vi "Dashboard Main.vi"() -> ()   [LabVIEW 2020]
uses:
  <vilib>/Utility/miscctls.llb/LVRowAndColumnTypeDef.ctl
  <vilib>/event_ctls.llb/eventvkey.ctl
  <vilib>/Rock Robotics/Network Tables/NT Read Numeric Array.vi
  <vilib>/Rock Robotics/Network Tables/NT Read Boolean.vi
  <vilib>/Rock Robotics/WPI/Dashboard/WPI_DashboardLogging Global.vi
panel:
  in  "Camera Settings Right":T1={"Frame Rate"=30, "Compression"=30, "Size"=1, "DB Camera Config"=FALSE} {"Frame Rate" scale=1.0..30.0; "Compression" scale=100.0..-1.0; "Size" items=["640x480", "320x240", "160x120"]}
  in  "Camera Name Right":string(combo)="No Camera Selection"
  out "Camera Perf":string
  in  "Camera Settings":T1={"Frame Rate"=30, "Compression"=30, "Size"=1, "DB Camera Config"=FALSE} {"Frame Rate" scale=1.0..30.0; "Compression" scale=100.0..-1.0; "Size" items=["640x480", "320x240", "160x120"]}
  in  "TCP":refnum<k5>
  in  "Rec Mode":enum32{"Stop", "Record", "Playback"}(radio)
  out "Robot IP":string
  out "Image Message":string="Timeout in Camera Communications"
  in  "Dashboard Tab":T2(tab)
  in  "Select Auto":string(combo)="Select Autonomous ..."
  out "NT Connection":bool
  out "MotorChart R":cluster{"Numeric":dbl, "Numeric":dbl}(graph)
  out "MotorChart L":cluster{"Numeric":dbl, "Numeric":dbl}(graph)
  out "MotorSliders R":cluster{"MotorSlide1":dbl, "MotorSlide2":dbl} {"MotorSlide2" scale=-1.0..1.0 scale format="%#_2e"; "MotorSlide1" scale=-1.0..1.0 scale format="%#_2e"}
  out "MotorSliders L":cluster{"MotorSlide1":dbl, "MotorSlide2":dbl} {"MotorSlide2" scale=-1.0..1.0 scale format="%#_2e"; "MotorSlide1" scale=-1.0..1.0 scale format="%#_2e"}
  out "Gyro":dbl(knob) scale=0.0..360.0
  out "JS1 Z":dbl(slide) scale=-1.0..1.0 scale format="%#_2e"
  out "JS1 Graph":cluster{"X":dbl, "Y":dbl}[](graph)
  out "JS1 Buttons":T3
  out "JS2 Z":dbl(slide) scale=-1.0..1.0 scale format="%#_2e"
  out "JS2 Graph":cluster{"X":dbl, "Y":dbl}[](graph)
  out "JS2 Buttons":T3
  out "Mode":T4(ring)=enum."Auto Disabled"
  out "Right Camera Perf":cluster{"Bandwidth (Mbps)":dbl, "FPS":dbl}
  out "Camera Image Right":T5(plugin-control)
  in  "DB/String 9":string
  in  "DB/String 8":string
  in  "DB/String 7":string
  in  "DB/String 6":string
  in  "DB/String 5":string
  in  "DB/String 4":string
  in  "DB/String 3":string
  in  "DB/String 2":string
  in  "DB/String 1":string
  in  "DB/String 0":string
  in  "DB/Slider 0":dbl(slide) scale=0.0..5.0
  in  "DB/Slider 1":dbl(slide) scale=0.0..5.0
  in  "DB/Slider 2":dbl(slide) scale=0.0..5.0
  in  "DB/Slider 3":dbl(slide) scale=0.0..5.0
  out "DB/LED 3":bool
  out "DB/LED 2":bool
  out "DB/LED 1":bool
  out "DB/LED 0":bool
  in  "DB/Button 3":bool
  in  "DB/Button 2":bool
  in  "DB/Button 1":bool
  in  "DB/Button 0":bool caption="New Name"
  out "Climb Time":dbl
  out "Current Shot":string
  out "Locked On":bool
  out "Ball Count":i32(slide) scale=0.0..2.0
  in  "Autonomous Selector":string(combo)
  in  "Test Slider":dbl(slide) scale=0.0..100.0 scale format="%#_3g"
  in  "On/Off":bool caption="Solenoid"
  in  "Test Name":u16(ring) items=["Select the test to run..."]
  in  "Test Tree":string(tree)
  in  "Motor":cluster{"Value":dbl, "Enable":bool} {"Value" scale=-1.0..1.0 scale format="%#_3g"}
  out "Progress":T6 {"Test Progress" scale=0.0..100.0}
  in  "Rev/Fwd":cluster{"Forward":bool, "Reverse":bool}
  in  "Test Ring":u16(ring) items=["Monochrome", "Color"]
  out "Cmd Status":string
  in  "Execute Command":bool
  in  "Command Params":string[][](table)
  in  "Command Selection":i32(listbox)
  in  "CheckList":i32(listbox)
  out "Tree":string(tree)
  out "Camera Image":T5(plugin-control)
  out "Background":bool
  in  "Camera Name":string(combo)="No Camera Selection"
  # "HW"
  # "HW"
  # "Joysticks"
  # "Drive Motors"
  # "Front"
  # "Right"
  # "Left"
  # "Back"
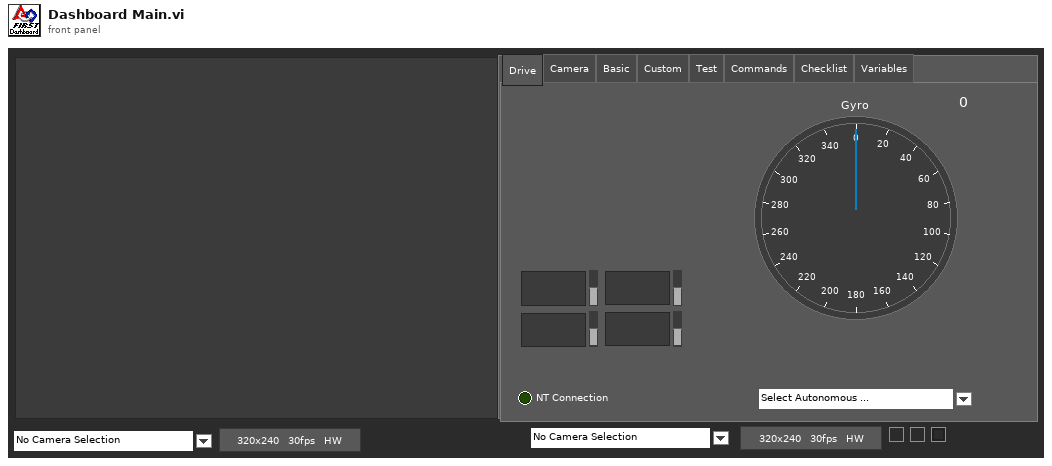
[diagram p1: front panel]
types:
  T1 = cluster{"Frame Rate":i32, "Compression":i32, "Size":u16, "DB Camera Config":bool}
  T2 = enum32{"Drive", "Camera", "Basic", "Custom", "Test", "Commands", "Checklist", "Variables"}
  T3 = cluster{bool, bool, bool, bool, bool, bool, bool, bool, bool, bool, bool, bool}
  T4 = enum8{"Tele-Op Disabled", "Tele-Op Enabled", "Auto Disabled", "Auto Enabled", "Test Disabled", "Test Enabled", "Disconnected", "No Code", "E-Stop"}
  T5 = typedef "IMAQ Image.ctl" = refnum<image>
  T6 = cluster{"Test Progress":u8, "Test Progress Text":string}
  T7 = cluster{"Save Path":path, "Interval (s)":dbl, "Keep":i32}
  T8 = typedef "Image Type" = u32
  T9 = cluster{"IDs":cluster{"RPC field ID":u16, "Unique ID":u16}, "String":string}
  T10 = cluster{"Error Strings":string, "Disable Counts":cluster{u16, u16}, "Rail Faults":cluster{u16, u16, u16}, "Robot IP":string, "DB Mode":u8, "Event Info":cluster{"Name":string, "Type":u8, "Number":u16, "Replay":u8}}
  T11 = cluster{"Storage":cluster{"Disk Free":u64, "RAM Block":u32, "RAM free":u32}, "CPU Utilization":cluster{"CPU % ISR":sgl, "CPU % Time Crit":sgl, "CPU % Timed Str":sgl, "CPU % High":sgl, "CPU % Above":sgl, "CPU % Normal":sgl, "CPU % Low":sgl}, "CAN":cluster{"% Bus Utilization":sgl, "Bus Off Cnt":u32, "TX_FIFO Full Cnt":u32, "Receive Error Cnt":u8, "Transmit Error Cnt":u8}, "HID":cluster{"HID Outputs":u32, "Rumble Low":u16, "Rumble High":u16}[]}
  T12 = cluster{"Status bits":cluster{"Test Mode":bool, "Autonomous":bool, "Enabled":bool, "Code Start":bool, "Brownout":bool, "Reserved 2":bool, "Reserved 3":bool, "E-Stop":bool}, "Code Trace":cluster{"Disabled":bool, "TeleOp":bool, "Auto":bool, "Test":bool}, "Controller Type":enum16{"unknown", "cRIO", "roboRio"}, "Code?":enum16{"unknown", "noCode", "code"}, "Battery V":dbl}
  T13 = cluster{"Control Bits":cluster{"TestMode":bool, "Autonomous":bool, "Enabled":bool, "FMS Present":bool, bool, bool, bool, "E-Stop":bool}, "Team Station ":u8, "Countdown":sgl, "Joystick Values":cluster{"Axes":dbl[], "Buttons":bool[], "POVs":i16[]}[]}
  T14 = cluster{"Axes":dbl[], "Buttons":bool[], "POVs":i16[]}[]
  T15 = cluster{"Axes":dbl[], "Buttons":bool[], "POVs":i16[]}
  T16 = cluster{"Buttons[0]":bool, "Buttons[1]":bool, "Buttons[2]":bool, "Buttons[3]":bool, "Buttons[4]":bool, "Buttons[5]":bool, "Buttons[6]":bool, "Buttons[7]":bool, "Buttons[8]":bool, "Buttons[9]":bool, "Buttons[10]":bool, "Buttons[11]":bool}
  T17 = cluster{"Camera Image":refnum<vi>, "Dashboard Tab":refnum<vi>, "Background":refnum<vi>, "Rec Mode":refnum<vi>, "Test Slider":refnum<vi>, "On/Off ":refnum<vi>, "Test Ring":refnum<vi>, "Rev/Fwd":refnum<vi>, "Test Name":refnum<vi>, "Motor":refnum<vi>, "Progress":refnum<vi>, "CheckList":refnum<vi>, "Tree":refnum<vi>, "Test Tree":refnum<vi>, "Command Params":refnum<vi>, "Command Selection":refnum<vi>, "Execute Command":refnum<vi>, "Cmd Status":refnum<vi>, "Camera Settings":refnum<vi>, "Camera Name":refnum<vi>, "Camera Perf":refnum<vi>, "Camera Settings Right":refnum<vi>, "Camera Name Right":refnum<vi>, "Camera Image Right":refnum<vi>}
  T18 = cluster{"Global Rectangle":i32[], "Contours":cluster{"Contour Type":u32, "ROI Type":u32, "Points":i32[]}[]}
  T19 = cluster{"Camera Name":string, string, "Saved DB Images Info":cluster{"Save Path":path, "Interval (s)":dbl, "Keep":i32}}
  T20 = cluster{"Camera Name Right":string, string, "Saved DB Images Info":cluster{"Save Path":path, "Interval (s)":dbl, "Keep":i32}}
  T21 = cluster{"Operation":enum16{"Update", "Clear"}, "Color Box":u32}[]
  T22 = typedef "eventvkey.ctl" = enum16{"ASCII", "Enter", "Return", "Shift", "Ctrl", "Alt", "Cmd", "Opt", "Caps", "NumLock", "Clear", "Break", "Up", "Down", "Left", "Right", "Insert", "Delete", "Home", "End", "PageUp", "PageDown", "Escape", "Help", "Pause", "ScrollLock", "F1", "F2", "F3", "F4", "F5", "F6", "F7", "F8", "F9", "F10", "F11", "F12", "F13", "F14", "F15", "F16", "F17", "F18", "F19", "F20", "F21", "F22", "F23", "F24", "Play", "VolumeUp", "VolumeDown", "Mute", "Two Byte Char"}
  T23 = cluster{"Image Size":bool, "Image Type":bool, "Pixel Value":bool, "ROI Information":bool, "Zoom Factor":bool}
  T24 = cluster{"Operation":enum16{"Update", "Clear"}, "Color Box":u32}
  T25 = typedef "LVRowAndColumnTypeDef.ctl" = cluster{"Row":i32, "Column":i32}
  T26 = cluster{"Shift":bool, "Ctrl":bool, "Alt":bool, "Cmd":bool, "Opt":bool}
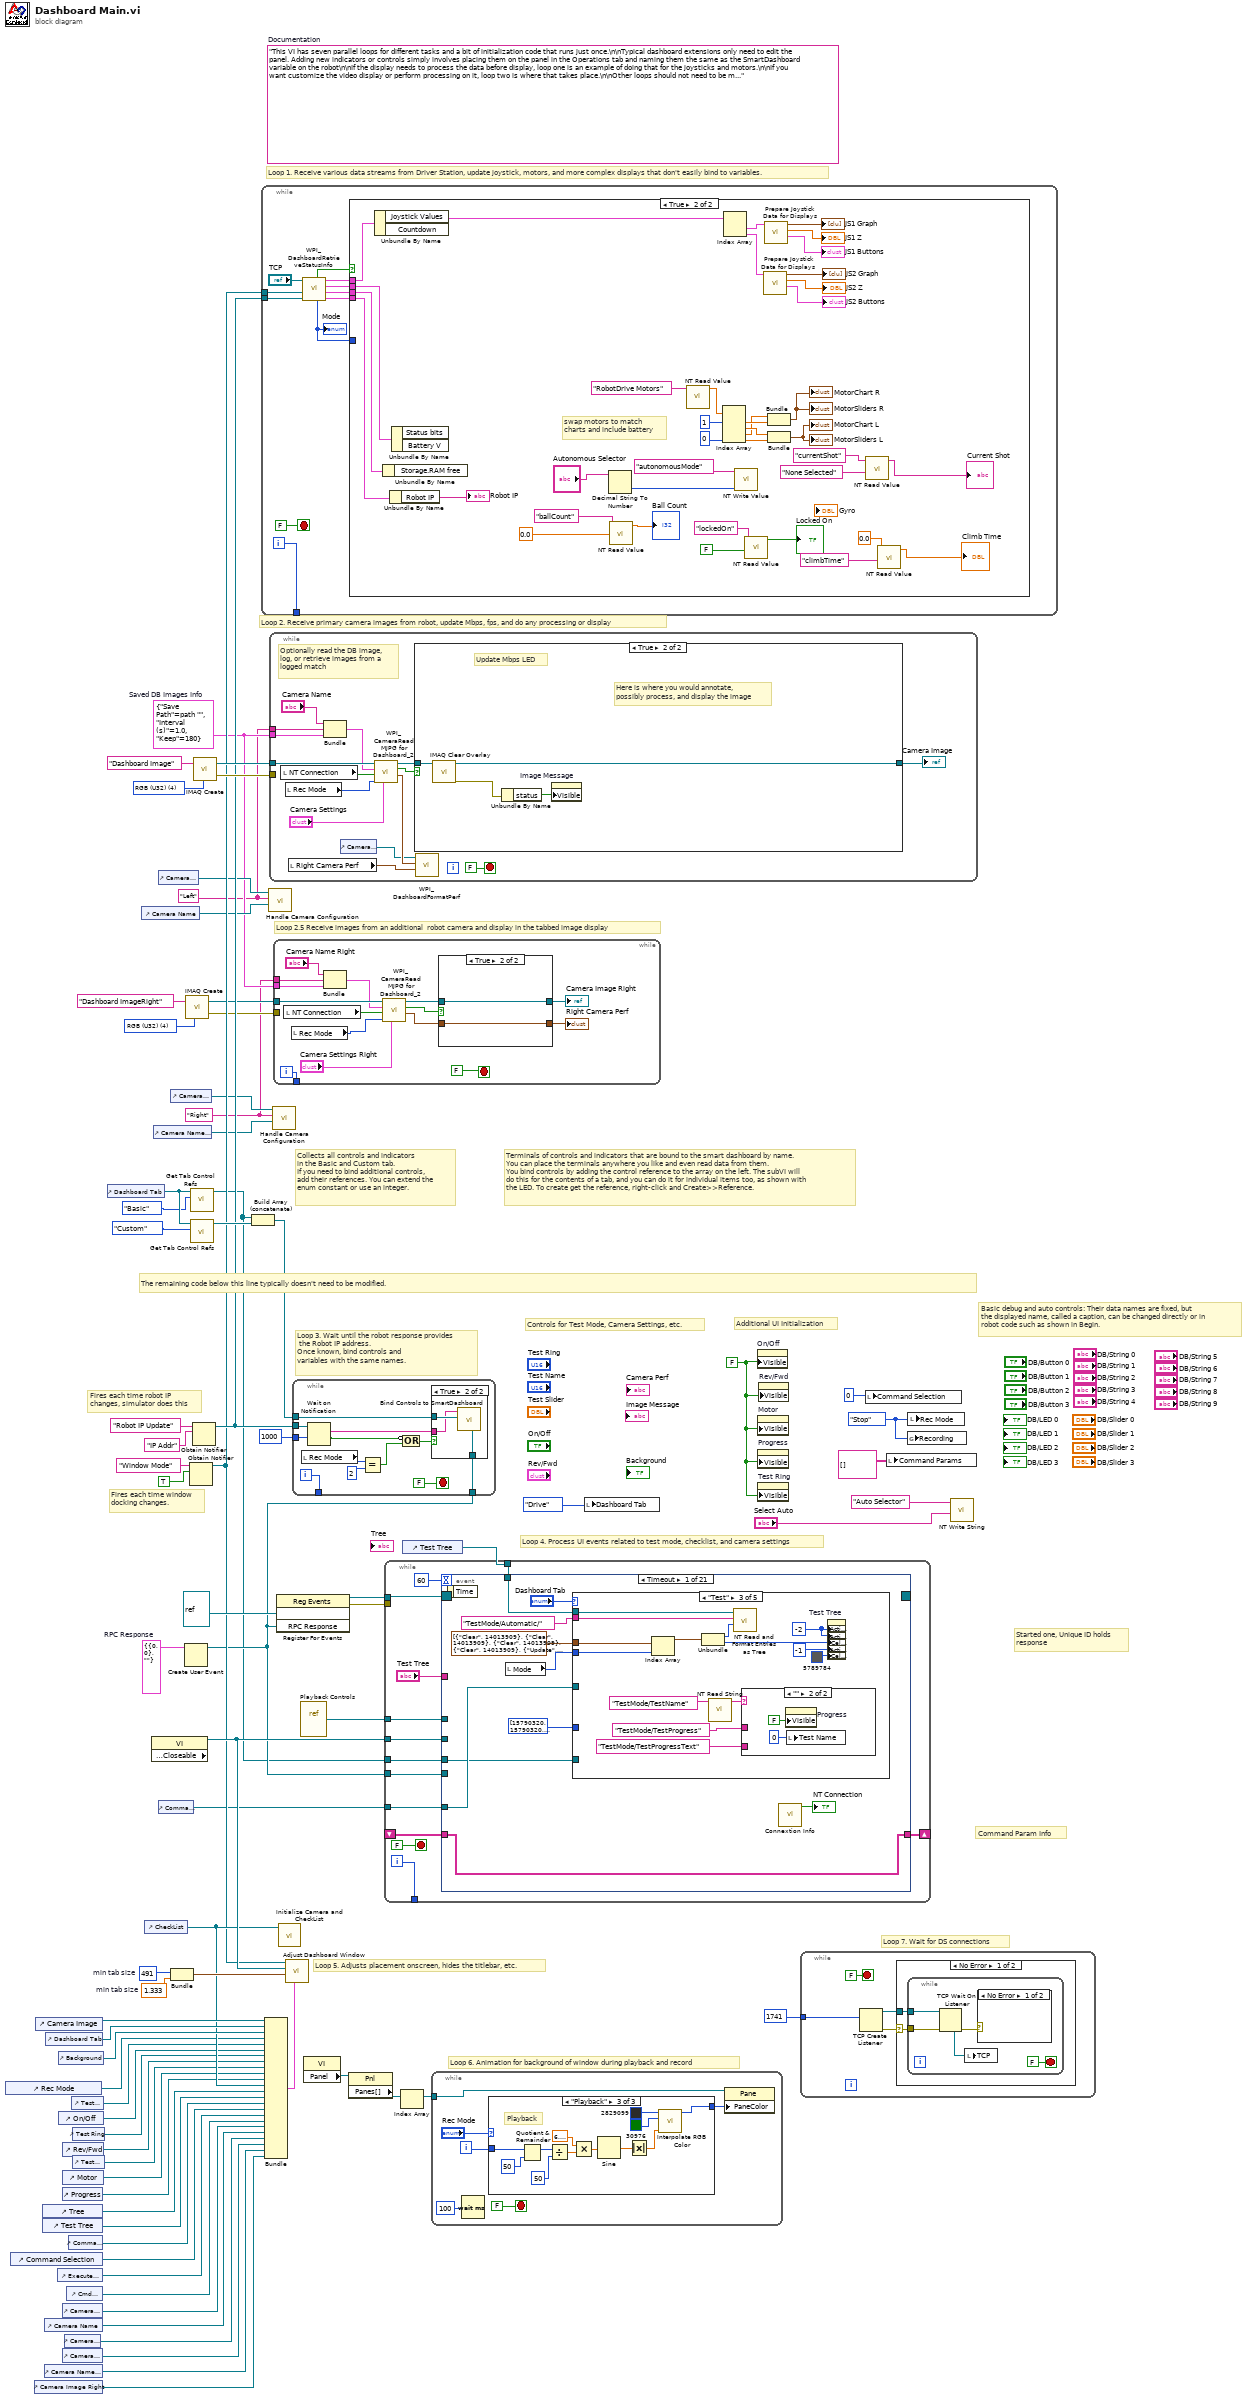
[diagram p0: block diagram]
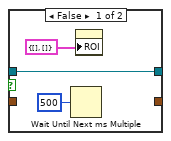
[diagram p2: hidden frame]
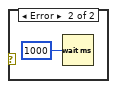
[diagram p3: hidden frame]
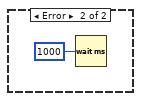
[diagram p4: hidden frame]
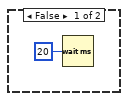
[diagram p5: hidden frame]
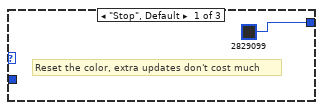
[diagram p6: hidden frame]
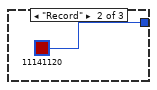
[diagram p7: hidden frame]
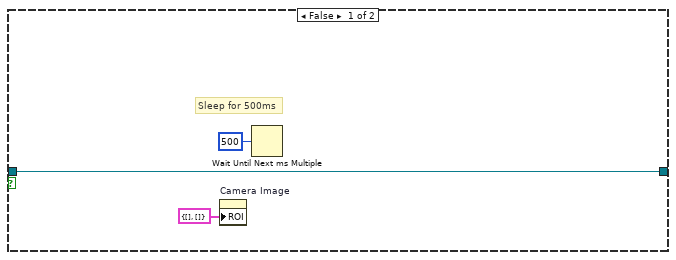
[diagram p9: hidden frame]
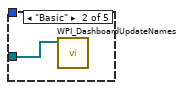
[diagram p11: hidden frame]
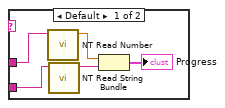
[diagram p12: hidden frame]
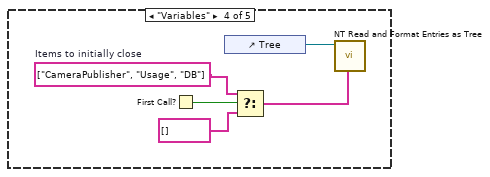
[diagram p13: hidden frame]
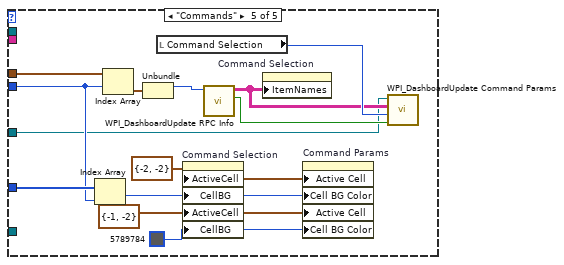
[diagram p14: hidden frame]
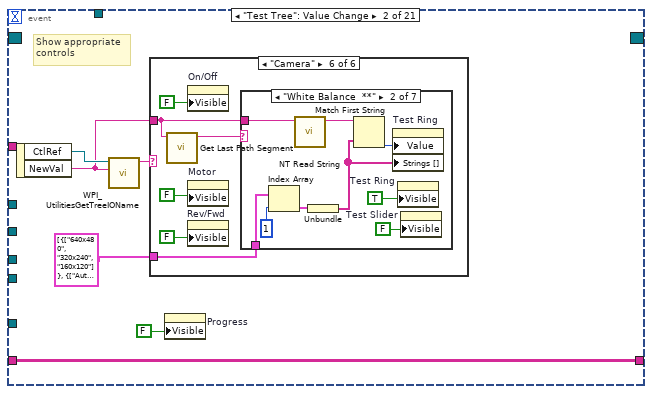
[diagram p15: hidden frame]
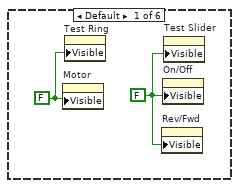
[diagram p16: hidden frame]
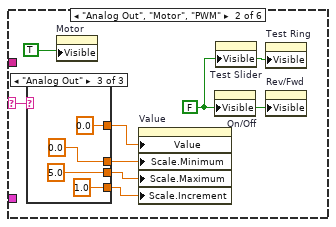
[diagram p17: hidden frame]
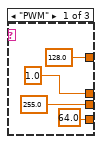
[diagram p18: hidden frame]
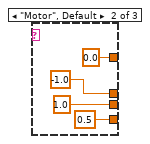
[diagram p19: hidden frame]
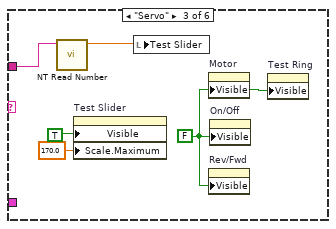
[diagram p20: hidden frame]
diagram:
  w3 = T7 {"Save Path"=path "", "Interval (s)"=1.0, "Keep"=180}  # Saved DB Images Info
  w2 = "Right"
  w1 = "Left"
  w13 = T8 4 items=["Grayscale (U8)", "Grayscale (I16)", "Grayscale (SGL)", "Complex (CSG)", "RGB (U32)", "HSL (U32)", "RGB (U64)"] ("Image Type")
  w29 = T9 {"IDs"={"RPC field ID"=0, "Unique ID"=0}, "String"=""}  # RPC Response
  w52 = 491  # min tab size
  w51 = 1.333  # min tab size
  w59 = enum32{"Stop", "Record", "Playback"}."Stop" ("Rec Mode")
  w36 = FALSE ("Visible")
  (unwired) "This VI has seven parallel loops for different tasks and a bit of initialization code that runs just once.\n\nTypical dashboard extensions only need to edit the panel. Adding new indicators or controls simply involves placing them on the panel in the Operations tab and naming them the same as the SmartDashboard variable on the robot\n\nIf the display needs to process the data before display, loop one is an example of doing that for the joysticks and motors.\n\nIf you want customize the video display or perform processing on it, loop two is where that takes place.\n\nOther loops should not need to be modified. They are pretty standard, and document the task they perform."  # Documentation
  w76 = T8 4 items=["Grayscale (U8)", "Grayscale (I16)", "Grayscale (SGL)", "Complex (CSG)", "RGB (U32)", "HSL (U32)", "RGB (U64)"] ("Image Type")
  # "Loop 2.5 Receive images from an additional  robot camera and display in the tabbed image display"
  # "Command Param Info"
  # "Started one, Unique ID holds\nresponse"
  # "Loop 7. Wait for DS connections"
  # "Basic debug and auto controls: Their data names are fixed, but\nthe displayed name, called a caption, can be changed directly or in\nrobot code such as shown in Begin."
  # "Controls for Test Mode, Camera Settings, etc."
  # "Additional UI Initialization"
  # "Loop 6. Animation for background of window during playback and record"
  # "Fires each time robot IP\nchanges, simulator does this"
  # "Fires each time window\ndocking changes."
  # "Collects all controls and indicators\nin the Basic and Custom tab.\nIf you need to bind additional controls,\nadd their references. You can extend the\nenum constant or use an integer."
  # "The remaining code below this line typically doesn't need to be modified."
  # "Loop 4. Process UI events related to test mode, checklist, and camera settings"
  # "Terminals of controls and indicators that are bound to the smart dashboard by name.\nYou can place the terminals anywhere you like and even read data from them.\nYou bind controls by adding the control reference to the array on the left. The subVI will\ndo this for the contents of a tab, and you can do it for individual items too, as shown with\nthe LED. To create get the reference, right-click and Create>>Reference."
  # "Loop 3. Wait until the robot response provides\n the Robot IP address.\nOnce known, bind controls and\nvariables with the same names."
  # "Loop 5. Adjusts placement onscreen, hides the titlebar, etc."
  # "Loop 1. Receive various data streams from Driver Station, update joystick, motors, and more complex displays that don't easily bind to variables."
  # "Loop 2. Receive primary camera images from robot, update Mbps, fps, and do any processing or display"
  n1 = control-ref of="Rec Mode"() -> (w42:refnum<vi>)
  n2 = control-ref of="Command Selection"() -> (w28:refnum<vi>)
  n3 = control-ref of="Camera Image Right"() -> (w6:refnum<vi>)
  n4 = control-ref of="Camera Image"() -> (w54:refnum<vi>)
  n5 = control-ref of="Tree"() -> (w46:refnum<vi>)
  n6 = control-ref of="Test Tree"() -> (w45:refnum<vi>)
  n7 = control-ref of="Camera Name"() -> (w19:refnum<vi>)
  n8 = control-ref of="Camera Name Right"() -> (w7:refnum<vi>)
  n9 = control-ref of="Dashboard Tab"() -> (w53:refnum<vi>)
  n10 = control-ref of="Execute Command"() -> (w30:refnum<vi>)
  n11 = control-ref of="Background"() -> (w49:refnum<vi>)
  n12 = control-ref of="On/Off"() -> (w40:refnum<vi>)
  n13 = control-ref of="Progress"() -> (w37:refnum<vi>)
  n14 = control-ref of="Camera Settings"() -> (w20:refnum<vi>)
  n15 = control-ref of="Camera Settings Right"() -> (w8:refnum<vi>)
  n16 = control-ref of="Rev/Fwd"() -> (w38:refnum<vi>)
  n17 = control-ref of="Motor"() -> (w43:refnum<vi>)
  n18 = control-ref of="Camera Perf"() -> (w18:refnum<vi>)
  n19 = control-ref of="Cmd Status"() -> (w24:refnum<vi>)
  n20 = control-ref of="Command Params"() -> (w31:refnum<vi>)
  n21 = control-ref of="Test Slider"() -> (w41:refnum<vi>)
  n22 = control-ref of="Test Ring"() -> (w39:refnum<vi>)
  n23 = control-ref of="Test Name"() -> (w44:refnum<vi>)
  n24 = control-ref of="Dashboard Tab"() -> (w57:refnum<vi>)
  n25 = control-ref of="Camera Name"() -> (w21:refnum<vi>)
  n26 = control-ref of="CheckList"() -> (w47:refnum<vi>)
  n27 = property class="VI" props=["Front Panel.Closeable"]() -> (reference out=w58:refnum<vi>)  [unwired: 2 in, 2 out]
  n28 = control-ref of="Camera Name Right"() -> (w9:refnum<vi>)
  n29 = control-ref of="Camera Settings"() -> (w22:refnum<vi>)
  n30 = control-ref of="Command Params"() -> (w23:refnum<vi>)
  n31 = control-ref of="Camera Settings Right"() -> (w10:refnum<vi>)
  n32 = Bundle("min tab size"=w52, "min tab size"=w51) -> (w50:cluster{"min tab size":i32, "min tab size":dbl})  [unwired: 1 in]
  n33 = Create User Event(user event datatype=w29) -> (user event=w25:refnum<user-event>)  [unwired: 1 in, 1 out]
  n34 = call "IMAQ Create"("Image Name"="Dashboard ImageRight", "Image Type"=w13) -> ("New Image"=w12:T5, "error out"=w11:errorcluster)  [unwired: 2 in, 1 out]
  n35 = Obtain Notifier(name (unnamed)="Window Mode", notification data type=TRUE) -> (notifier out=w34:refnum<notifier>)  [unwired: 2 in, 2 out]
  n36 = call <vilib>:"Get Tab Control Refs.vi"("Page Index"=T2."Basic" ("Dashboard Tab"), "TabControl in"=w57) -> ("ControlsOnPage"=w17:refnum<vi>[])  [unwired: 9 in]
  n37 = call <vilib>:"Get Tab Control Refs.vi"("Page Index"=T2."Custom" ("Dashboard Tab"), "TabControl in"=w57) -> ("ControlsOnPage"=w56:refnum<vi>[])  [unwired: 9 in]
  n38 = Obtain Notifier(name (unnamed)="Robot IP Update", notification data type="IP Addr" ("name (unnamed)")) -> (notifier out=w35:refnum<notifier>)  [unwired: 2 in, 2 out]
  n39 = call "IMAQ Create"("Image Name"="Dashboard Image", "Image Type"=w76) -> ("New Image"=w74:T5, "error out"=w73:errorcluster)  [unwired: 2 in, 1 out]
  n40 = Build Array (concatenate)(w17, w56) -> (w55:refnum<vi>[])
  n41 = while {
    tunnel: [w86] -> _
    tunnel: w35 -> [w80]
    tunnel: w34 -> [w77]
    i -> [w86]
    stop <- FALSE stop-if-true
    n42 = call <vilib>:"WPI_DashboardRetrieveStatusInfo.vi"("Binding Refnum"=w80, "Window Mode Notifier"=w77, "TCP Cnx"="TCP") -> ("Power and Errors"=w81:T10, "Robot Metrics"=w84:T11, "Status Info"=w85:T12, "Control Info"=w82:T13, "Robot Mode"=w79:T4, "Process?"=w83:bool)  [unwired: 3 in]
    "Mode" <- w79
    n43 = case shown="True" w83 {
      tunnel: w85 -> [_ w127]
      tunnel: w84 -> [_ w126]
      tunnel: w82 -> [_ w125]
      tunnel: w81 -> [_ w124]
      tunnel: w79 -> [_ _]
      frame False {
        n44 = Wait (ms)(milliseconds to wait=u32 20) -> ()  [unwired: 1 out]
      }
      frame True {
        # "swap motors to match\ncharts and include battery"
        n45 = Unbundle By Name(w125) -> ("Joystick Values"=w115:T14)  [unwired: 1 out]
        n46 = Unbundle By Name(w126) -> ()  [unwired: 1 out]
        n47 = Unbundle By Name(w124) -> ("Robot IP"=→"Robot IP":string)
        n48 = Unbundle By Name(w127) -> ()  [unwired: 2 out]
        n49 = Decimal String To Number(string="Autonomous Selector") -> (number=w102:i32)  [unwired: 2 in, 1 out]
        n50 = call-poly <vilib>:"NT Read Value.vi"("Default Value"=0.0, "Name"="ballCount") -> ("Numeric"=→"Ball Count":dbl)  [unwired: 8 in, 1 out]
        n51 = call-poly <vilib>:"NT Read Value.vi"("Name"="RobotDrive Motors") -> ("Numeric Array"=w105:dbl[])  [unwired: 9 in, 1 out]
        n52 = Index Array(array=w105, index #1=1, index #4=0) -> (element #1=w119:dbl, element #2=w120:dbl, element #3=w118:dbl, element #4=w123:dbl)  [unwired: 2 in]
        n53 = Index Array(array=w115) -> (element #1=w114:T15, element #2=w110:T15)  [unwired: 2 in]
        n54 = call-poly <vilib>:"NT Write Value.vi"("Numeric"=w102, "Name"="autonomousMode") -> ()  [unwired: 9 in, 1 out]
        n55 = call-poly <vilib>:"NT Read Value.vi"("Default Value"=FALSE, "Name"="lockedOn") -> ("Boolean"=→"Locked On":bool)  [unwired: 8 in, 1 out]
        n56 = call "Prepare Joystick Data for Displays.vi"("Joystick Values"=w110) -> ("Buttons"=→"JS2 Buttons":T16, "Z Axis"=→"JS2 Z":dbl, "Cartesian Data"=→"JS2 Graph":cluster{"X axis":dbl, "X axis":dbl}[])  [unwired: 8 in]
        n57 = call "Prepare Joystick Data for Displays.vi"("Joystick Values"=w114) -> ("Buttons"=→"JS1 Buttons":T16, "Z Axis"=→"JS1 Z":dbl, "Cartesian Data"=→"JS1 Graph":cluster{"X axis":dbl, "X axis":dbl}[])  [unwired: 8 in]
        n58 = Bundle("Numeric"=w118, "Numeric"=w119) -> (→"MotorChart R" →"MotorSliders R":cluster{"Numeric":dbl, "Numeric":dbl})  [unwired: 1 in]
        n59 = Bundle("Numeric"=w120, "Numeric"=w123) -> (→"MotorChart L" →"MotorSliders L":cluster{"Numeric":dbl, "Numeric":dbl})  [unwired: 1 in]
        n60 = call-poly <vilib>:"NT Read Value.vi"("Default Value"="None Selected", "Name"="currentShot") -> ("String"=→"Current Shot":string)  [unwired: 8 in, 1 out]
        n61 = call-poly <vilib>:"NT Read Value.vi"("Default Value"=0.0, "Name"="climbTime") -> ("Numeric"=→"Climb Time":dbl)  [unwired: 8 in, 1 out]
      }
    }
  }
  n62 = Bundle("Camera Image"=w54, "Dashboard Tab"=w53, "Background"=w49, "Rec Mode"=w42, "Test Slider"=w41, "On/Off"=w40, "Test Ring"=w39, "Rev/Fwd"=w38, "Test Name"=w44, "Motor"=w43, "Progress"=w37, "CheckList"=w47, "Tree"=w46, "Test Tree"=w45, "Command Params"=w31, "Command Selection"=w28, "Execute Command"=w30, "Cmd Status"=w24, "Camera Settings"=w20, "Camera Name"=w19, "Camera Perf"=w18, "Camera Settings Right"=w8, "Camera Name Right"=w7, "Camera Image Right"=w6) -> (w48:T17)  [unwired: 1 in]
  n63 = call "Handle Camera Configuration.vi"("CameraNameRef"=w21, "Display Name"=w1, "ClusterRef"=w22) -> ()  [unwired: 9 in]
  n64 = while {
    tunnel: w74 -> [w141]
    tunnel: w73 -> [_]
    tunnel: w3 -> [w134]
    tunnel: w1 -> [w131]
    stop <- FALSE stop-if-true
    # "Optionally read the DB image,\nlog, or retrieve images from a\nlogged match"
    n65 = local read "NT Connection"() -> (w135:bool)
    n66 = local read "Rec Mode"() -> (w138:enum32{"Stop", "Record", "Playback"})
    n67 = local read "Right Camera Perf"() -> (w129:cluster{"Bandwidth (Mbps)":dbl, "FPS":dbl})
    n68 = Bundle("Camera Name"="Camera Name", w131, "Saved DB Images Info"=w134) -> (w133:T19)  [unwired: 1 in]
    n69 = control-ref of="Camera Perf"() -> (w128:refnum<vi>)
    n70 = call <vilib>:"WPI_CameraRead MJPG for Dashboard_2.vi"("Camera Settings"="Camera Settings", "Rec Mode"=w138, "NT Connection"=w135, "Capture Info"=w133, "Image in"=w141) -> ("perf info"=w130:cluster{"Bandwidth (Mbps)":dbl, "fps":dbl}, "Active"=w139:bool, "Image\\ out"=w140:T5)  [unwired: 4 in]
    n71 = case shown="True" w139 {
      tunnel: w140 -> [w144 w147]
      tunnel: [w144 w146] -> w136
      frame False {
        # "Sleep for 500ms"
        n72 = property on="Camera Image" class="ImageControl"("ROI"=T18 {"Global Rectangle"=[], "Contours"=[]}) -> ()  [unwired: 2 in, 2 out]
        n73 = Wait Until Next ms Multiple(millisecond multiple=u32 500) -> ()  [unwired: 1 out]
      }
      frame True {
        # "Here is where you would annotate,\npossibly process, and display the image"
        # "Update Mbps LED"
        n74 = call "IMAQ Clear Overlay"("Image"=w147) -> ("error out"=w148:errorcluster, "Image Out"=w146:T5)  [unwired: 2 in, 7 out]
        n75 = Unbundle By Name(w148) -> ("status"=w149:bool)
        n76 = property on="Image Message" class="Str"("Visible"=w149) -> ()  [unwired: 2 in, 2 out]
      }
    }
    "Camera Image" <- w136
    n77 = call <vilib>:"WPI_DashboardFormatPerf.vi"("Right Camera Perf"=w129, "Performance"=w130, "String in"=w128) -> ()  [unwired: 9 in]
  }
  n78 = call "Handle Camera Configuration.vi"("CameraNameRef"=w9, "Display Name"=w2, "ClusterRef"=w10) -> ()  [unwired: 9 in]
  n79 = while {
    tunnel: w12 -> [w164]
    tunnel: w11 -> [_]
    tunnel: [w159] -> _
    tunnel: w3 -> [w155]
    tunnel: w2 -> [w152]
    i -> [w159]
    stop <- FALSE stop-if-true
    n80 = local read "NT Connection"() -> (w156:bool)
    n81 = local read "Rec Mode"() -> (w163:enum32{"Stop", "Record", "Playback"})
    n82 = Bundle("Camera Name Right"="Camera Name Right", w152, "Saved DB Images Info"=w155) -> (w154:T20)  [unwired: 1 in]
    n83 = call <vilib>:"WPI_CameraRead MJPG for Dashboard_2.vi"("Camera Settings"="Camera Settings Right", "Rec Mode"=w163, "NT Connection"=w156, "Capture Info"=w154, "Image in"=w164) -> ("perf info"=w150:cluster{"Bandwidth (Mbps)":dbl, "fps":dbl}, "Active"=w158:bool, "Image\\ out"=w161:T5)  [unwired: 4 in]
    n84 = case shown="True" w158 {
      tunnel: w161 -> [w166 w169]
      tunnel: [w166 w169] -> w157
      tunnel: [_ w168] -> w151
      tunnel: w150 -> [_ w168]
      frame False {
        n85 = Wait Until Next ms Multiple(millisecond multiple=u32 500) -> ()  [unwired: 1 out]
        n86 = property on="Camera Image Right" class="ImageControl"("ROI"=T18 {"Global Rectangle"=[], "Contours"=[]}) -> ()  [unwired: 2 in, 2 out]
      }
      frame True {
      }
    }
    "Camera Image Right" <- w157
    "Right Camera Perf" <- w151
  }
  n87 = register-events(refnum<vi> refnum, w25) -> (reference out=w63:refnum<event-registration>, error out=w62:errorcluster)  [unwired: 2 in]
  n88 = call "Initialize Camera and CheckList.vi"("ListBox in"=w47) -> ()  [unwired: 11 in]
  n89 = call "Adjust Dashboard Window.vi"("Sizing Refnums"=w48, "Size Constraints"=w50, "VI"=w58, "WIn Mode"=w34) -> ()  [unwired: 8 in]
  n90 = while {
    tunnel: w55 -> [w181]
    tunnel: w35 -> [w179]
    tunnel: [w177] -> _
    tunnel: u32 1000 ("milliseconds to wait") -> [w176]
    tunnel: w25 -> [w170]
    i -> [w177]
    stop <- FALSE stop-if-true
    n91 = local read "Rec Mode"() -> (w172:enum32{"Stop", "Record", "Playback"})
    n92 = Wait on Notification(notifier=w179, timeout in ms (-1)=w176) -> (notification=w178:string, timed out?=w174:bool)  [unwired: 2 in, 2 out]
    n93 = Equal?(x=w172, y=u16 2 ("Rec Mode")) -> (x = y?=w173:bool)
    n94 = Compound Arithmetic op=OR(invert w174, w173) -> (w175:bool)
    n95 = case shown="True" w175 {
      tunnel: w181 -> [_ w184]
      tunnel: w178 -> [_ w183]
      tunnel: w170 -> [_ w182]
      frame False {
      }
      frame True {
        n96 = call <vilib>:"Bind Controls to SmartDashboard.vi"("RPC ref"=w182, "Bound Control Refs"=w184, "Server IP Address"=w183) -> ()  [unwired: 9 in]
      }
    }
  }
  n97 = vi-ref "Playback Controls.vi"() -> (w64:refnum<vi>)
  n98 = property class="VI"() -> ("Panel"=w66:refnum<vi>)  [unwired: 2 in, 2 out]
  n99 = property class="Pnl"(reference=w66) -> ("Panes[]"=w67:refnum<vi>[])  [unwired: 1 in, 2 out]
  n100 = Index Array(array=w67) -> (element=w65:refnum<vi>)  [unwired: 1 in]
  n101 = control-ref of="Test Tree"() -> (w68:refnum<vi>)
  n102 = while {
    tunnel: [w194] -> _
    tunnel: w68 -> [w193]
    tunnel: w64 -> [w192]
    tunnel: w63 -> [w191]
    tunnel: w62 -> [_]
    tunnel: w58 -> [w190]
    tunnel: w25 -> [w189]
    tunnel: w23 -> [w188]
    shift-right: [w187] -> _
    shift-left: _ -> [w186]
    tunnel: w17 -> [w185]
    i -> [w194]
    stop <- FALSE stop-if-true
    n103 = event shown="[0] Timeout" {
      selector: w191 -> [_ _ _ _ _ _ _ _ _ _ _ _ _ _ _ _ _ _ _ _ _]
      dyn-events: [_ _ _ _ _ _ _ _ _ _ _ _ _ _ _ _ w454 _ _ _ _] -> _
      timeout: u32 60 ("milliseconds to wait") -> [_ _ _ _ _ _ _ _ _ _ _ _ _ _ _ _ _ _ _ _ _]
      tunnel: w193 -> [w206 _ _ _ _ _ _ _ _ _ _ _ _ _ _ _ _ _ _ _ _]
      tunnel: "Test Tree" -> [_ _ _ _ _ _ _ _ _ _ _ w421 w429 w431 w435 w443 _ _ _ _ _]
      tunnel: w192 -> [_ _ _ _ _ _ _ _ _ _ _ _ _ _ _ _ w456 _ w474 _ _]
      tunnel: w190 -> [_ _ _ _ _ _ _ _ _ _ _ _ _ _ _ _ w452 _ _ _ _]
      tunnel: w189 -> [_ _ _ _ _ _ _ _ _ _ _ _ _ _ _ _ w450 _ _ _ _]
      tunnel: w188 -> [w201 _ _ _ _ _ w372 _ _ _ _ _ _ _ _ _ _ _ _ _ _]
      tunnel: [w200 w249 w351 w356 w365 w369 w370 w379 w389 w396 w408 w420 w427 w430 w434 w442 w449 w469 w471 w475 w488] -> w187
      tunnel: w186 -> [w200 w249 w351 w356 w365 w369 w370 _ _ w396 w408 w420 w427 w430 w434 w442 w449 w469 w471 w475 w488]
      tunnel: w185 -> [w198 _ _ _ _ _ _ _ _ _ _ _ _ _ _ _ _ _ _ _ _]
      event Timeout {
        n104 = event-data() -> ()  [unwired: 1 in, 1 out]
        n105 = local read "Mode"() -> (w203:T4)
        n106 = case shown="\"Test\"" "Dashboard Tab" {
          tunnel: w206 -> [_ _ w222 _ _]
          tunnel: "TestMode/Automatic/" ("Name Pattern") -> [_ _ w221 _ _]
          tunnel: T21 [{"Operation"=enum."Clear", "Color Box"=14013909}, {"Operation"=enum."Clear", "Color Box"=14013909}, {"Operation"=enum."Clear", "Color Box"=14013909}, {"Operation"=enum."Clear", "Color Box"=14013909}, {"Operation"=enum."Update", "Color Box"=14013909}, {"Operation"=enum."Update", "Color Box"=16777215}, {"Operation"=enum."Clear", "Color Box"=14013909}, {"Operation"=enum."Clear", "Color Box"=14013909}, {"Operation"=enum."Clear", "Color Box"=14013909}] -> [_ _ w214 _ w242]
          tunnel: w203 -> [_ _ w213 _ w241]
          tunnel: u32[] [15790320, 15790320, 15790320, 15790320, 16777215, 16777215, 15790320, 15790320, 15790320] -> [_ _ _ _ w247]
          tunnel: w201 -> [_ _ _ _ w235]
          tunnel: w198 -> [_ w208 _ _ _]
          frame "Custom", Default {
          }
          frame "Basic" {
            n107 = call <vilib>:"WPI_DashboardUpdateNames.vi"("Controls on Tab"=w208) -> ()  [unwired: 11 in]
          }
          frame "Test" {
            w220 = -2 ("Active Item:Row Number")
            n108 = Index Array(array=w214, index=w213) -> (element=w215:T24)
            n109 = Unbundle(w215) -> ("Operation"=w216:enum16{"Update", "Clear"}, "Color Box"=w217:u32)
            n110 = call <vilib>:"NT Read String.vi"("Name"="TestMode/TestName") -> ("String"=w211:string)  [unwired: 9 in, 1 out]
            n111 = call <vilib>:"NT Read and Format Entries as Tree.vi"("Operation"=w216, "Name Pattern"=w221, "Tree Refnum"=w222) -> ()  [unwired: 7 in, 2 out]
            n112 = case shown="\"\"" w211 {
              tunnel: "TestMode/TestProgress" ("Name") -> [w224 _]
              tunnel: "TestMode/TestProgressText" ("Name") -> [w223 _]
              frame Default {
                n113 = call <vilib>:"NT Read Number.vi"("Name"=w224) -> ("Numeric"=w225:dbl)  [unwired: 9 in, 1 out]
                n114 = call <vilib>:"NT Read String.vi"("Name"=w223) -> ("String"=w226:string)  [unwired: 9 in, 1 out]
                n115 = Bundle("Numeric"=w225, "String"=w226) -> (→"Progress":cluster{"Numeric":dbl, "String":string})  [unwired: 1 in]
              }
              frame "" {
                n116 = property on="Progress" class="Clust (strict)"("Visible"=FALSE) -> ()  [unwired: 2 in, 2 out]
                n117 = local write "Test Name"(u16 0) -> ()
              }
            }
            n118 = property on="Test Tree" class="Tree (strict)"("Active Item Row Number"=w220, "ActiveColNum"=w220, "CellBG"=w217, "Active Item Row Number"=-1 ("Active Item:Row Number"), "CellBG"=u32 5789784 ("Color Box")) -> ()  [unwired: 2 in, 2 out]
          }
          frame "Variables" {
            w232 = string[] ["CameraPublisher", "Usage", "DB"]  # Items to initially close
            n119 = First Call?() -> (First Call?: T/F=w233:bool)
            n120 = control-ref of="Tree"() -> (w234:refnum<vi>)
            n121 = Select(t=w232, s=w233, f=string[] []) -> (s? t:f=w230:string[])
            n122 = call <vilib>:"NT Read and Format Entries as Tree.vi"("Tags to  Close"=w230, "Tree Refnum"=w234) -> ()  [unwired: 8 in, 2 out]
          }
          frame "Commands" {
            w243 = u32 5789784 ("Color Box")
            w244 = T25 {"Row"=-1, "Column"=-2} ("Active Cell:Active Cell")
            w246 = T25 {"Row"=-2, "Column"=-2} ("Active Cell:Active Cell")
            n123 = Index Array(array=w247, index=w241) -> (element=w245:u32)
            n124 = Index Array(array=w242, index=w241) -> (element=w240:T24)
            n125 = Unbundle(w240) -> ("Operation"=w239:enum16{"Update", "Clear"})  [unwired: 1 out]
            n126 = local read "Command Selection"() -> (w238:i32)
            n127 = property on="Command Selection" class="MCListbox (strict)"("ActiveCell"=w246, "CellBG"=w245, "ActiveCell"=w244, "CellBG"=w243) -> ()  [unwired: 2 in, 2 out]
            n128 = call <vilib>:"WPI_DashboardUpdate RPC Info.vi"("Operation"=w239) -> ("update"=w237:bool, "commands"=w236:string[][])  [unwired: 9 in]
            n129 = property on="Command Selection" class="MCListbox (strict)"("ItemNames"=w236) -> ()  [unwired: 2 in, 2 out]
            n130 = property on="Command Params" class="Tbl (strict)"("Active Cell"=w246, "Cell BG Color"=w245, "Active Cell"=w244, "Cell BG Color"=w243) -> ()  [unwired: 2 in, 2 out]
            n131 = call <vilib>:"WPI_DashboardUpdate Command Params.vi"("Update"=w237, "NewVal"=w238, "Commands"=w236, "Param Tbl"=w235) -> ()  [unwired: 7 in, 1 out]
          }
        }
        n132 = call <vilib>:"Connextion Info.vi"() -> ("Connected"=→"NT Connection":bool)  [unwired: 10 in, 1 out]
      }
      event "Test Tree": Value Change {
        # "Show appropriate\ncontrols"
        n133 = event-data() -> ("CtlRef"=w252:refnum<vi>, "NewVal"=w250:string)  [unwired: 1 in]
        n134 = call <vilib>:"WPI_UtilitiesGetTreeIOName.vi"("NewVal"=w250, "TreeControl in"=w252) -> ("I/O Name"=w253:string)  [unwired: 9 in]
        n135 = case shown="\"Camera\"" w253 {
          selector: w253 -> [_ w260 _ w282 w291 _]
          tunnel: w250 -> [_ _ w279 w281 _ w298]
          tunnel: cluster{string[]}[] [{["640x480", "320x240", "160x120"]}, {["Auto", "Fixed indoor", "Fixed outdoor 1", "Fixed outdoor 2", "Fixed fluorescent 1", "Fixed fluorescent 2", "Hold current"]}, {["Auto", "Flicker-free 50 Hz", "Flicker-free 60 Hz", "Hold current"]}, {["None", "Prioritize frame rate", "Prioritize image quality"]}, {["Monochrome", "Color"]}] -> [_ _ _ _ _ w297]
          frame Default {
            w255 = FALSE ("Visible")
            w254 = FALSE ("Visible")
            n136 = property on="Motor" class="Clust (strict)"("Visible"=w254) -> ()  [unwired: 2 in, 2 out]
            n137 = property on="Test Ring" class="Ring (strict)"("Visible"=w254) -> ()  [unwired: 2 in, 2 out]
            n138 = property on="Rev/Fwd" class="Clust (strict)"("Visible"=w255) -> ()  [unwired: 2 in, 2 out]
            n139 = property on="On/Off" class="Bool (strict)"("Visible"=w255) -> ()  [unwired: 2 in, 2 out]
            n140 = property on="Test Slider" class="Slide (strict)"("Visible"=w255) -> ()  [unwired: 2 in, 2 out]
          }
          frame "Analog Out", "Motor", "PWM" {
            w261 = FALSE ("Visible")
            n141 = case shown="\"Analog Out\"" w260 {
              tunnel: [1.0 ("Value") -1.0 ("Value") 0.0 ("Value")] -> w259
              tunnel: [255.0 ("Value") 1.0 ("Value") 5.0 ("Value")] -> w258
              tunnel: [128.0 ("Value") 0.0 ("Value") 0.0 ("Value")] -> w257
              tunnel: [64.0 ("Value") 0.5 ("Value") 1.0 ("Value")] -> w256
              frame "PWM" {
              }
              frame "Motor", Default {
              }
              frame "Analog Out" {
              }
            }
            n142 = property on="Motor" class="Clust (strict)"("Visible"=TRUE) -> ()  [unwired: 2 in, 2 out]
            n143 = property on="Value" class="Slide (strict)"("Value"=w257, "Scale.Minimum"=w259, "Scale.Maximum"=w258, "Scale.Increment"=w256) -> ()  [unwired: 2 in, 2 out]
            n144 = property on="On/Off" class="Bool (strict)"("Visible"=w261) -> ()  [unwired: 2 in, 2 out]
            n145 = property on="Test Slider" class="Slide (strict)"("Visible"=w261) -> ()  [unwired: 2 in, 2 out]
            n146 = property on="Test Ring" class="Ring (strict)"("Visible"=w261) -> ()  [unwired: 2 in, 2 out]
            n147 = property on="Rev/Fwd" class="Clust (strict)"("Visible"=w261) -> ()  [unwired: 2 in, 2 out]
          }
          frame "Servo" {
            w277 = FALSE ("Visible")
            n148 = call <vilib>:"NT Read Number.vi"("Name"=w279) -> ("Numeric"=w278:dbl)  [unwired: 9 in, 1 out]
            n149 = property on="Test Slider" class="Slide (strict)"("Visible"=TRUE, "Scale.Maximum"=170.0 ("Scale.Range:Maximum")) -> ()  [unwired: 2 in, 2 out]
            n150 = local write "Test Slider"(w278) -> ()
            n151 = property on="Motor" class="Clust (strict)"("Visible"=w277) -> ()  [unwired: 2 in, 2 out]
            n152 = property on="Rev/Fwd" class="Clust (strict)"("Visible"=w277) -> ()  [unwired: 2 in, 2 out]
            n153 = property on="On/Off" class="Bool (strict)"("Visible"=w277) -> ()  [unwired: 2 in, 2 out]
            n154 = property on="Test Ring" class="Ring (strict)"("Visible"=w277) -> ()  [unwired: 2 in, 2 out]
          }
          frame "Relay", "Solenoid" {
            w280 = FALSE ("Visible")
            n155 = property on="Motor" class="Clust (strict)"("Visible"=w280) -> ()  [unwired: 2 in, 2 out]
            n156 = property on="Test Slider" class="Slide (strict)"("Visible"=w280) -> ()  [unwired: 2 in, 2 out]
            n157 = Search and Replace String(input string=w281, search string="/Value  **", replace string="/Direction") -> (result string=w287:string)  [unwired: 5 in, 3 out]
            n158 = property on="Test Ring" class="Ring (strict)"("Visible"=w280) -> ()  [unwired: 2 in, 2 out]
            n159 = call <vilib>:"NT Read String.vi"("Name"=w287) -> ("String"=w285:string)  [unwired: 9 in, 1 out]
            n160 = Equal?(x="Both directions", y=w285) -> (x = y?=w283:bool)
            n161 = Not(x=w283) -> (.not. x?=w284:bool)
            n162 = property on="Rev/Fwd" class="Clust (strict)"("Visible"=w283) -> ()  [unwired: 2 in, 2 out]
            n163 = property on="On/Off" class="Bool (strict)"("Visible"=w284, "Caption.Text"=w282) -> ()  [unwired: 2 in, 2 out]
          }
          frame "Compressor", "Digital Out" {
            w290 = FALSE ("Visible")
            # "Get direction and finish"
            n164 = property on="Motor" class="Clust (strict)"("Visible"=w290) -> ()  [unwired: 2 in, 2 out]
            n165 = property on="Test Slider" class="Slide (strict)"("Visible"=w290) -> ()  [unwired: 2 in, 2 out]
            n166 = property on="Test Ring" class="Ring (strict)"("Visible"=w290) -> ()  [unwired: 2 in, 2 out]
            n167 = property on="On/Off" class="Bool (strict)"("Visible"=TRUE, "Caption.Text"=w291) -> ()  [unwired: 2 in, 2 out]
            n168 = property on="Rev/Fwd" class="Clust (strict)"("Visible"=FALSE) -> ()  [unwired: 2 in, 2 out]
          }
          frame "Camera" {
            n169 = call <vilib>:"Get Last Path Segment.vi"("String in"=w298) -> ("String out"=w299:string)  [unwired: 10 in]
            n170 = property on="On/Off" class="Bool (strict)"("Visible"=FALSE) -> ()  [unwired: 2 in, 2 out]
            n171 = property on="Motor" class="Clust (strict)"("Visible"=FALSE) -> ()  [unwired: 2 in, 2 out]
            n172 = property on="Rev/Fwd" class="Clust (strict)"("Visible"=FALSE) -> ()  [unwired: 2 in, 2 out]
            n173 = case shown="\"White Balance  **\"" w299 {
              tunnel: w298 -> [w305 w314 w323 w332 w341 _ w347]
              tunnel: w297 -> [w303 w311 w320 w329 w338 _ _]
              frame "Size  **" {
                n174 = Index Array(array=w303) -> (element=w302:cluster{string[]})  [unwired: 1 in]
                n175 = call <vilib>:"NT Read String.vi"("Name"=w305) -> ("String"=w304:string)  [unwired: 9 in, 1 out]
                n176 = Unbundle(w302) -> (w300:string[])
                n177 = Match First String(2:w300, 3:w304) -> (0:w301:i32)  [unwired: 1 out]
                n178 = property on="Test Ring" class="Ring (strict)"("Value"=w301, "Strings []"=w300) -> ()  [unwired: 2 in, 2 out]
                n179 = property on="Test Ring" class="Ring (strict)"("Visible"=TRUE) -> ()  [unwired: 2 in, 2 out]
                n180 = property on="Test Slider" class="Slide (strict)"("Visible"=FALSE) -> ()  [unwired: 2 in, 2 out]
              }
              frame "White Balance  **" {
                n181 = Index Array(array=w311, index=1) -> (element=w312:cluster{string[]})
                n182 = call <vilib>:"NT Read String.vi"("Name"=w314) -> ("String"=w313:string)  [unwired: 9 in, 1 out]
                n183 = Unbundle(w312) -> (w309:string[])
                n184 = Match First String(2:w309, 3:w313) -> (0:w308:i32)  [unwired: 1 out]
                n185 = property on="Test Ring" class="Ring (strict)"("Value"=w308, "Strings []"=w309) -> ()  [unwired: 2 in, 2 out]
                n186 = property on="Test Ring" class="Ring (strict)"("Visible"=TRUE) -> ()  [unwired: 2 in, 2 out]
                n187 = property on="Test Slider" class="Slide (strict)"("Visible"=FALSE) -> ()  [unwired: 2 in, 2 out]
              }
              frame "Exposure  **" {
                n188 = Index Array(array=w320, index=2) -> (element=w321:cluster{string[]})
                n189 = call <vilib>:"NT Read String.vi"("Name"=w323) -> ("String"=w322:string)  [unwired: 9 in, 1 out]
                n190 = Unbundle(w321) -> (w317:string[])
                n191 = Match First String(2:w317, 3:w322) -> (0:w318:i32)  [unwired: 1 out]
                n192 = property on="Test Ring" class="Ring (strict)"("Value"=w318, "Strings []"=w317) -> ()  [unwired: 2 in, 2 out]
                n193 = property on="Test Ring" class="Ring (strict)"("Visible"=TRUE) -> ()  [unwired: 2 in, 2 out]
                n194 = property on="Test Slider" class="Slide (strict)"("Visible"=FALSE) -> ()  [unwired: 2 in, 2 out]
              }
              frame "Exposure Priority  **" {
                n195 = Index Array(array=w329, index=3) -> (element=w330:cluster{string[]})
                n196 = call <vilib>:"NT Read String.vi"("Name"=w332) -> ("String"=w331:string)  [unwired: 9 in, 1 out]
                n197 = Unbundle(w330) -> (w326:string[])
                n198 = Match First String(2:w326, 3:w331) -> (0:w327:i32)  [unwired: 1 out]
                n199 = property on="Test Ring" class="Ring (strict)"("Value"=w327, "Strings []"=w326) -> ()  [unwired: 2 in, 2 out]
                n200 = property on="Test Ring" class="Ring (strict)"("Visible"=TRUE) -> ()  [unwired: 2 in, 2 out]
                n201 = property on="Test Slider" class="Slide (strict)"("Visible"=FALSE) -> ()  [unwired: 2 in, 2 out]
              }
              frame "Color Enable  **" {
                n202 = Index Array(array=w338, index=4) -> (element=w339:cluster{string[]})
                n203 = call <vilib>:"NT Read String.vi"("Name"=w341) -> ("String"=w340:string)  [unwired: 9 in, 1 out]
                n204 = Unbundle(w339) -> (w335:string[])
                n205 = Match First String(2:w335, 3:w340) -> (0:w336:i32)  [unwired: 1 out]
                n206 = property on="Test Ring" class="Ring (strict)"("Value"=w336, "Strings []"=w335) -> ()  [unwired: 2 in, 2 out]
                n207 = property on="Test Ring" class="Ring (strict)"("Visible"=TRUE) -> ()  [unwired: 2 in, 2 out]
                n208 = property on="Test Slider" class="Slide (strict)"("Visible"=FALSE) -> ()  [unwired: 2 in, 2 out]
              }
              frame Default {
                n209 = property on="Test Ring" class="Ring (strict)"("Visible"=FALSE) -> ()  [unwired: 2 in, 2 out]
                n210 = property on="Test Slider" class="Slide (strict)"("Visible"=FALSE) -> ()  [unwired: 2 in, 2 out]
              }
              frame "Brightness  **", "Color Level  **", "Compression  **", "FPS  **", "Sharpness  **" {
                n211 = call <vilib>:"NT Read Number.vi"("Name"=w347) -> ("Numeric"=w346:dbl)  [unwired: 9 in, 1 out]
                n212 = local write "Test Slider"(w346) -> ()
                n213 = property on="Test Slider" class="Slide (strict)"("Visible"=TRUE, "Scale.Maximum"=100.0 ("Scale.Range:Maximum")) -> ()  [unwired: 2 in, 2 out]
                n214 = property on="Test Ring" class="Ring (strict)"("Visible"=FALSE) -> ()  [unwired: 2 in, 2 out]
              }
            }
          }
        }
        n215 = property on="Progress" class="Clust (strict)"("Visible"=FALSE) -> ()  [unwired: 2 in, 2 out]
      }
      event "Test Name": Mouse Enter {
        # "Populate the ring with the list of tests"
        n216 = event-data() -> ()  [unwired: 1 in, 1 out]
        n217 = call <vilib>:"NT Read String Array.vi"("Name"="TestMode/TestList") -> ("String Array"=w355:string[])  [unwired: 9 in, 1 out]
        n218 = Build Array (concatenate)("Select the test to run...", w355) -> (w354:string[])
        n219 = property on="Test Name" class="Ring (strict)"("Strings []"=w354) -> ()  [unwired: 2 in, 2 out]
      }
      event "Test Name": Value Change {
        w357 = FALSE ("Visible")
        # "Tell the robot the test name to run"
        n220 = event-data() -> ("NewVal"=w361:u16)  [unwired: 1 in]
        n221 = property on="Test Name" class="Ring (strict)"() -> ("Strings []"=w362:string[])  [unwired: 2 in, 2 out]
        n222 = local write "Progress"(T6 {"Test Progress"=0, "Test Progress Text"=""} ("Progress")) -> ()
        n223 = Index Array(array=w362, index=w361) -> (element=w360:string)
        n224 = call <vilib>:"NT Write String.vi"("String"=w360, "Name"="TestMode/TestName") -> ()  [unwired: 9 in, 1 out]
        n225 = property on="Progress" class="Clust (strict)"("Visible"=TRUE) -> ()  [unwired: 2 in, 2 out]
        n226 = property on="Motor" class="Clust (strict)"("Visible"=w357) -> ()  [unwired: 2 in, 2 out]
        n227 = property on="Test Slider" class="Slide (strict)"("Visible"=w357) -> ()  [unwired: 2 in, 2 out]
        n228 = property on="On/Off" class="Bool (strict)"("Visible"=w357) -> ()  [unwired: 2 in, 2 out]
        n229 = property on="Rev/Fwd" class="Clust (strict)"("Visible"=w357) -> ()  [unwired: 2 in, 2 out]
        n230 = property on="Test Ring" class="Ring (strict)"("Visible"=w357) -> ()  [unwired: 2 in, 2 out]
      }
      event "Select Auto": Mouse Enter {
        # "Populate the combo box with the list of autonomous options"
        n231 = event-data() -> ()  [unwired: 1 in, 1 out]
        n232 = call <vilib>:"NT Read String Array.vi"("Name"="Auto List") -> ("String Array"=w364:string[])  [unwired: 9 in, 1 out]
        n233 = property on="Select Auto" class="CmbBox"("Strings[]"=w364) -> ()  [unwired: 2 in, 2 out]
      }
      event "Select Auto": Value Change {
        # "User modified the Auto Selection. Write to NT variable so robot knows."
        n234 = event-data() -> ("NewVal"=w367:string)  [unwired: 1 in]
        n235 = call <vilib>:"NT Write String.vi"("String"=w367, "Name"="Auto Selector") -> ()  [unwired: 9 in, 1 out]
      }
      event "Command Selection": Value Change {
        # "Get the params and show in table"
        n236 = event-data() -> ("NewVal"=w373:i32)  [unwired: 1 in]
        n237 = property on="Command Selection" class="MCListbox (strict)"() -> ("ItemNames"=w371:string[][])  [unwired: 2 in, 2 out]
        n238 = call <vilib>:"WPI_DashboardUpdate Command Params.vi"("NewVal"=w373, "Commands"=w371, "Param Tbl"=w372) -> ()  [unwired: 8 in, 1 out]
      }
      event "Execute Command": Value Change {
        # "Started one, Unique ID holds\nresponse"
        n239 = event-data() -> ()  [unwired: 1 in, 1 out]
        n240 = property on="Command Selection" class="MCListbox (strict)"() -> ("ItemNames"=w384:string[][])  [unwired: 2 in, 2 out]
        n241 = Index Array(array=w384, index (row)="Command Selection", index (col)=0) -> (element=w382:string)
        n242 = call <vilib>:"Invoke Commands.vi"("Command Params"="Command Params", "Function Name"=w382) -> ("Params"=w378:u8, "Started"=w377:bool)  [unwired: 7 in, 1 out]
        n243 = Array Subset(array="Command Params", length (row)=w378) -> (w379:string[][])  [unwired: 3 in]
        n244 = Select(t="Executing" ("Cmd Status"), s=w377, f="" ("Cmd Status")) -> (s? t:f=→"Cmd Status":string)
      }
      event "Command Selection": Double Click {
        n245 = event-data() -> ("Row"=w392:i32)  [unwired: 1 in]
        n246 = property on="Command Selection" class="MCListbox (strict)"() -> ("ItemNames"=w395:string[][])  [unwired: 2 in, 2 out]
        n247 = local read "Command Params"() -> (w391:string[][])
        n248 = Index Array(array=w395, index (row)=w392, index (col)=0) -> (element=w393:string)
        n249 = call <vilib>:"Invoke Commands.vi"("Command Params"=w391, "Function Name"=w393) -> ("Params"=w390:u8, "Started"=w385:bool)  [unwired: 7 in, 1 out]
        n250 = Array Subset(array=w391, length (row)=w390) -> (w389:string[][])  [unwired: 3 in]
        n251 = Select(t="Executing" ("Cmd Status"), s=w385, f="" ("Cmd Status")) -> (s? t:f=w386:string)
        n252 = local write "Cmd Status"(w386) -> ()
      }
      event "CheckList": Double Click {
        # "Shift clears all"
        # "Update symbols on the listbox"
        n253 = event-data() -> ("PlatMods.Shift"=w397:bool, "Row"=w399:i32)  [unwired: 1 in]
        n254 = case shown="True" w397 {
          tunnel: w399 -> [w403 _]
          tunnel: 1 -> [w402 _]
          frame False {
            n255 = property on="CheckList" class="LstBox (strict)"() -> ("Item Symbols"=w401:i32[])  [unwired: 2 in, 2 out]
            n256 = Replace Array Subset(array=w401, new element=w402, index=w403) -> (w400:i32[])
            n257 = property on="CheckList" class="LstBox (strict)"("Item Symbols"=w400) -> ()  [unwired: 2 in, 2 out]
          }
          frame True {
            w404 = 0 ("Top Row")
            n258 = property on="CheckList" class="LstBox (strict)"() -> ("Number of Rows"=w406:u32)  [unwired: 2 in, 2 out]
            n259 = Initialize Array(0, w406) -> (w405:i32[])
            n260 = property on="CheckList" class="LstBox (strict)"("Top Row"=w404, "Value"=w404, "Item Symbols"=w405) -> ()  [unwired: 2 in, 2 out]
          }
        }
      }
      event "CheckList": Key Down {
        # "Update symbols on the listbox\nLeft and right keys check and uncheck"
        n261 = event-data() -> ("VKey"=w410:T22)  [unwired: 1 in]
        n262 = case shown="\"Left\", \"Right\"" w410 {
          selector: w410 -> [w415 _]
          tunnel: eventvkey."Left" ("VKey") -> [w413 _]
          frame "Left", "Right" {
            n263 = Equal?(x=w413, y=w415) -> (x = y?=w414:bool)
            n264 = Select(t=0, s=w414, f=1) -> (s? t:f=w416:i32)
            n265 = property on="CheckList" class="LstBox (strict)"() -> ("Item Symbols"=w419:i32[])  [unwired: 2 in, 2 out]
            n266 = Replace Array Subset(array=w419, new element=w416, index="CheckList") -> (w418:i32[])
            n267 = property on="CheckList" class="LstBox (strict)"("Item Symbols"=w418) -> ()  [unwired: 2 in, 2 out]
          }
          frame Default {
          }
        }
      }
      event "Motor.Enable": Value Change {
        # "When the test mode otor enable helper is set, update that\ntree row item's value"
        n268 = event-data() -> ("NewVal"=w425:bool)  [unwired: 1 in]
        n269 = Unbundle("Motor") -> ("Value"=w424:dbl)  [unwired: 1 out]
        n270 = Select(t=w424, s=w425, f=0.0) -> (s? t:f=w422:dbl)
        n271 = call <vilib>:"NT Write Number.vi"("Numeric"=w422, "Name"=w421) -> ()  [unwired: 9 in, 1 out]
      }
      event "Test Slider": Value Change {
        # "When the test mode slider helper is set, update that\ntree row item's value"
        n272 = event-data() -> ("NewVal"=w428:dbl)  [unwired: 1 in]
        n273 = call <vilib>:"NT Write Number.vi"("Numeric"=w428, "Name"=w429) -> ()  [unwired: 9 in, 1 out]
      }
      event "On/Off": Value Change {
        # "When the test mode on/off helper value is set, update that\ntree row item's value"
        n274 = event-data() -> ("NewVal"=w433:bool)  [unwired: 1 in]
        n275 = Boolean To (0,1)(Boolean=w433) -> (0, 1=w432:i16)
        n276 = call <vilib>:"NT Write Number.vi"("Numeric"=w432, "Name"=w431) -> ()  [unwired: 9 in, 1 out]
      }
      event "Rev/Fwd": Value Change {
        # "When the test mode helper value for relays is set, update that\ntree row item's value"
        n277 = event-data() -> ("NewVal.Forward"=w441:bool, "NewVal.Reverse"=w440:bool)  [unwired: 1 in]
        n278 = Boolean To (0,1)(Boolean=w441) -> (0, 1=w437:i16)
        n279 = Boolean To (0,1)(Boolean=w440) -> (0, 1=w439:i16)
        n280 = Negate(x=w439) -> (-x=w438:i16)
        n281 = Add(x=w437, y=w438) -> (x+y=w436:i16)
        n282 = call <vilib>:"NT Write Number.vi"("Numeric"=w436, "Name"=w435) -> ()  [unwired: 9 in, 1 out]
      }
      event "Test Ring": Value Change {
        # "When a test mode helper value is selected from the ring,\nset the tree item's variable to the string value"
        n283 = event-data() -> ("NewVal"=w445:u16)  [unwired: 1 in]
        n284 = property on="Test Ring" class="Ring (strict)"() -> ("Strings []"=w446:string[])  [unwired: 2 in, 2 out]
        n285 = Index Array(array=w446, index=w445) -> (element=w444:string)
        n286 = call <vilib>:"NT Write String.vi"("String"=w444, "Name"=w443) -> ()  [unwired: 9 in, 1 out]
      }
      event "Rec Mode": Value Change {
        # "Update globals for recording mode and path to read log from.\nClear when logging and let NetworkTables set path for vision to\nuse."
        n287 = event-data() -> ("NewVal"=w457:enum32{"Stop", "Record", "Playback"})  [unwired: 1 in]
        n288 = global write "WPI_DashboardLogging Global.vi" "Logging Filename"(path "") -> ()
        n289 = global write "WPI_DashboardLogging Global.vi" "Recording"(w457) -> ()
        n290 = case shown="\"Playback\"" w457 {
          tunnel: w456 -> [_ w459 w468]
          tunnel: [_ _ w467] -> w454
          tunnel: [_ _ w466] -> _
          tunnel: w452 -> [_ _ w464]
          tunnel: cluster{i32, i32} {-250, 170} -> [_ _ w463]
          tunnel: [_ _ T23 {"Image Size"=TRUE, "Image Type"=TRUE, "Pixel Value"=TRUE, "ROI Information"=TRUE, "Zoom Factor"=FALSE} ("Image Information Shown:All Elements")] -> w447
          tunnel: [_ _ TRUE ("Zoom Factor")] -> w448
          tunnel: w450 -> [_ _ w460]
          frame Default {
          }
          frame "Stop", "Record" {
            # "Place Window too"
            n291 = invoke class="VI" method="FP.Close"(reference=w459) -> (reference out=w458:refnum<vi>)  [unwired: 2 in, 2 out]
            n292 = invoke class="VI" method="Abort VI"(reference=w458) -> ()  [unwired: 2 in, 3 out]
          }
          frame "Playback" {
            n293 = call "Open Playback Panel.vi"("Offset"=w463, "DB VI Ref"=w464, "Playback in"=w468) -> ("Playback out"=w465:refnum<vi>)  [unwired: 8 in]
            n294 = register-events(w465, w460) -> (reference out=w467:refnum<event-registration>, error out=w466:errorcluster)  [unwired: 2 in]
          }
        }
        n295 = property on="Camera Image Right" class="ImageControl"("Image Information Shown"=w447, "Image Information Visible"=w448) -> ()  [unwired: 2 in, 2 out]
        n296 = property on="Camera Image" class="ImageControl"("Image Information Shown"=w447, "Image Information Visible"=w448) -> ()  [unwired: 2 in, 2 out]
        n297 = call <vilib>:"WPI_DashboardNT Log FieldName Cache.vi"("Operation"=enum16{"Lookup/Add", "Index", "Clear"}."Clear") -> ()  [unwired: 8 in, 3 out]
      }
      event Panel Close {
        w470 = enum32{"Stop", "Record", "Playback"}."Stop" ("Rec Mode")
        # "Playback window has been closed, abort"
        n298 = event-data() -> ()  [unwired: 1 in, 4 out]
        n299 = local write "Rec Mode"(w470) -> ()
        n300 = global write "WPI_DashboardLogging Global.vi" "Recording"(w470) -> ()
      }
      event Panel Close {
        # "Abort playback window and ourself"
        n301 = event-data() -> ()  [unwired: 1 in, 4 out]
        n302 = invoke class="VI" method="FP.Close"(reference=w474) -> (reference out=w473:refnum<vi>)  [unwired: 2 in, 2 out]
        n303 = invoke class="VI" method="Abort VI"(reference=w473) -> (error out=w472:errorcluster)  [unwired: 2 in, 2 out]
        n304 = invoke class="VI" method="Abort VI"(error in=w472) -> ()  [unwired: 2 in, 3 out]
      }
      event User Event {
        n305 = event-data() -> ("IDs"=w481:cluster{"RPC field ID":u16, "Unique ID":u16}, "String"=w480:string)  [unwired: 1 in]
        n306 = Bundle("IDs"=w481, "String"=w480) -> (w479:T9)  [unwired: 1 in]
        n307 = call <vilib>:"Retrieve RPC Response.vi"("RPC Response"=w479) -> ("Output"=w477:string[][])  [unwired: 10 in]
        n308 = Build Array (concatenate)(w475, w477) -> (w476:string[][])
        n309 = local write "Command Params"(w476) -> ()
        n310 = local write "Cmd Status"("" ("Cmd Status")) -> ()
      }
      event "Tree": Double Click {
        n311 = event-data() -> ("PlatMods"=w487:T26, "Tag"=w484:string)  [unwired: 1 in]
        n312 = Unbundle(w487) -> ("Shift"=w486:bool)  [unwired: 4 out]
        n313 = String Subset(string=w484, length (rest)=1 ("length (rest)")) -> (substring=w483:string)  [unwired: 1 in]
        n314 = Not(x=w486) -> (.not. x?=w485:bool)
        n315 = case shown="\"/\"" w483 {
          tunnel: w484 -> [_ w490]
          tunnel: w485 -> [_ w489]
          frame Default {
          }
          frame "/" {
            n316 = call <vilib>:"NT Update Persistence.vi"("Persistence"=w489, "Name"=w490) -> ()  [unwired: 9 in, 1 out]
          }
        }
      }
    }
  }
  n317 = while {
    tunnel: w65 -> [w492]
    i -> [w495]
    stop <- FALSE stop-if-true
    n318 = Wait (ms)(milliseconds to wait=u32 100) -> ()  [unwired: 1 out]
    n319 = case shown="\"Playback\"" "Rec Mode" {
      tunnel: w495 -> [_ _ w510]
      tunnel: [u32 2829099 ("Base Color") u32 11141120 ("Target Color") w499] -> w491
      frame "Stop", Default {
        # "Reset the color, extra updates don't cost much"
      }
      frame "Record" {
      }
      frame "Playback" {
        # "Playback"
        n320 = Quotient & Remainder(x=w510, y=u32 50 ("milliseconds to wait")) -> (x-y*floor(x/y)=w506:u32)  [unwired: 1 out]
        n321 = Divide(x=w506, y=u32 50 ("milliseconds to wait")) -> (x/y=w503:dbl)
        n322 = Multiply(x=6.283185307179586, y=w503) -> (x*y=w508:dbl)
        n323 = Sine(x=w508) -> (sin(x)=w507:dbl)
        n324 = Absolute Value(x=w507) -> (abs(x)=w500:dbl)
        n325 = call "Interpolate RGB Color.vi"("Proportion"=w500, "Target Color"=u32 30976, "Base Color"=u32 2829099) -> ("Result Color"=w499:u32)  [unwired: 8 in]
      }
    }
    n326 = property class="Pane"(reference=w492, "PaneColor"=w491) -> ()  [unwired: 1 in, 2 out]
  }
  n327 = local write "Dashboard Tab"(T2."Drive" ("Dashboard Tab")) -> ()
  n328 = property on="On/Off" class="Bool (strict)"("Visible"=w36) -> ()  [unwired: 2 in, 2 out]
  n329 = property on="Motor" class="Clust (strict)"("Visible"=w36) -> ()  [unwired: 2 in, 2 out]
  n330 = property on="Progress" class="Clust (strict)"("Visible"=w36) -> ()  [unwired: 2 in, 2 out]
  n331 = property on="Test Ring" class="Ring (strict)"("Visible"=w36) -> ()  [unwired: 2 in, 2 out]
  n332 = property on="Rev/Fwd" class="Clust (strict)"("Visible"=w36) -> ()  [unwired: 2 in, 2 out]
  n333 = while {
    tunnel: u16 1741 ("timeout ms (25000)") -> [w512]
    stop <- FALSE stop-if-true
    n334 = TCP Create Listener(10:w512) -> (0:w511:errorcluster, 3:w513:refnum<k5>)  [unwired: 4 in, 1 out]
    n335 = case shown="No Error" w511 {
      selector: w511 -> [w515 _]
      tunnel: w513 -> [w516 _]
      frame No Error {
        n336 = while {
          tunnel: w516 -> [w519]
          tunnel: w515 -> [w518]
          stop <- FALSE stop-if-true
          n337 = TCP Wait On Listener(8:w518, 11:w519) -> (0:w520:errorcluster, 4:w521:refnum<k5>)  [unwired: 2 in, 3 out]
          n338 = local write "TCP"(w521) -> ()
          n339 = case shown="No Error" w520 {
            frame No Error {
            }
            frame Error {
              n340 = Wait (ms)(milliseconds to wait=u32 1000) -> ()  [unwired: 1 out]
            }
          }
        }
      }
      frame Error {
        n341 = Wait (ms)(milliseconds to wait=u32 1000) -> ()  [unwired: 1 out]
      }
    }
  }
  n342 = local write "Command Selection"(u16 0 ("milliseconds to wait")) -> ()
  n343 = local write "Command Params"(string[][] [] ("Command Params")) -> ()
  n344 = global write "WPI_DashboardLogging Global.vi" "Recording"(w59) -> ()
  n345 = local write "Rec Mode"(w59) -> ()
  n346 = call <vilib>:"NT Write String.vi"("String"="Select Auto", "Name"="Auto Selector") -> ()  [unwired: 9 in, 1 out]
